vi "INTELLIFAUCET Ready-NotReady.vi"(4 "Refnum in":T1, 6 "Debug":bool, 8 "Error In":errorcluster, 10 "READY?":enum8{"READY", "NOT READY"}(ring), 11 "VISA session":refnum<visa-resource-name>="MW100") -> (0 "Error Out":errorcluster, 3 "dup VISA session":refnum<visa-resource-name>)   [LabVIEW 2016]
uses:
  MW100/Type Definitions/HEWH MW100 Channel Numbers.ctl
  Type Definitions/HEWH Normally Open Valve Control.ctl
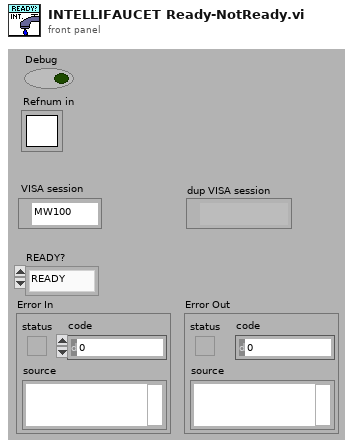
[diagram p1: front panel]
types:
  T1 = typedef "Semaphore RefNum" = refnum<k1>
  T2 = typedef "HEWH MW100 Channel Numbers.ctl" = string
  T3 = typedef "HEWH Normally Open Valve Control.ctl" = string
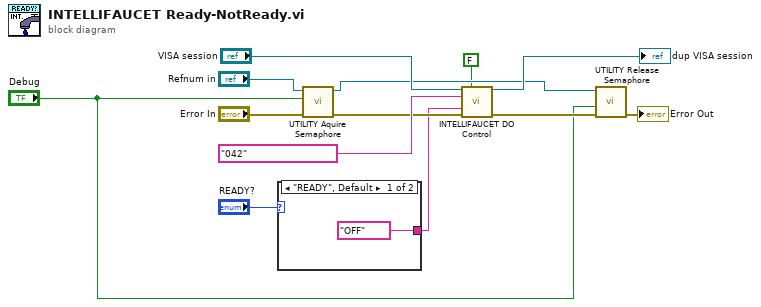
[diagram p0: block diagram]
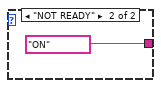
[diagram p2: hidden frame]
diagram:
  n1 = case shown="\"READY\", Default" "READY?" {
    tunnel: [T3 "OFF" ("Normally Open Valve") T3 "ON" ("Normally Open Valve")] -> w1
    frame "READY", Default {
    }
    frame "NOT READY" {
    }
  }
  n2 = call "UTILITY Aquire Semaphore.vi"("error in (no error)"="Error In", "Debug"="Debug", "Refnum in"="Refnum in") -> ("error out"=w8:errorcluster, "Refnum out"=w5:T1)  [unwired: 6 in, 1 out]
  n3 = call "INTELLIFAUCET DO Control.vi"("VISA session"="VISA session", "Normally Closed Valve?"=FALSE, "HEWH MW100 Channel Numbers"=T2 "042", "Normally Open Valve"=w1, "Error In"=w8) -> ("dup VISA session"=→"dup VISA session":refnum<visa-resource-name>, "error out"=w7:errorcluster)  [unwired: 7 in, 2 out]
  n4 = call "UTILITY Release Semaphore.vi"("error in (no error)"=w7, "Debug"="Debug", "Refnum in"=w5) -> ("error out"=→"Error Out":errorcluster)  [unwired: 8 in]
